vi "S2DS_Scan type change.vi"(10 "All channel parameters":T1 {"Scan parameters"."Y data taking" items=["in both direction", "in up direction only", "in down direction only"]; "Scan parameters"."X data taking" items=["in both direction", "in up direction only", "in down direction only"]}) -> (2 "All channel parameters (out)":T1 {"Scan parameters"."Y data taking" items=["in both direction", "in up direction only", "in down direction only"]; "Scan parameters"."X data taking" items=["in both direction", "in up direction only", "in down direction only"]})   [LabVIEW 2025]
uses:
  TYPE DEFS/S2DS_All Channel Parameters.ctl
  TYPE DEFS/S2DS_WC info.ctl
  TYPE DEFS/S2DS_Single WC info.ctl
  TYPE DEFS/S2DS_RC info.ctl
  TYPE DEFS/S2DS_Single RC info.ctl
  TYPE DEFS/S2DS_DAC info new.ctl
  TYPE DEFS/S2DS_Single DC info.ctl
  TYPE DEFS/S2DS_Array Inst Info.ctl
  TYPE DEFS/S2DS_Sweep Info.ctl
panel:
  out "String":string
  in  "Select Y channel":u16(ring) items=["A", "B"]
  in  "Select X channel":u16(ring) items=["A", "B"]
  in  "stop":bool
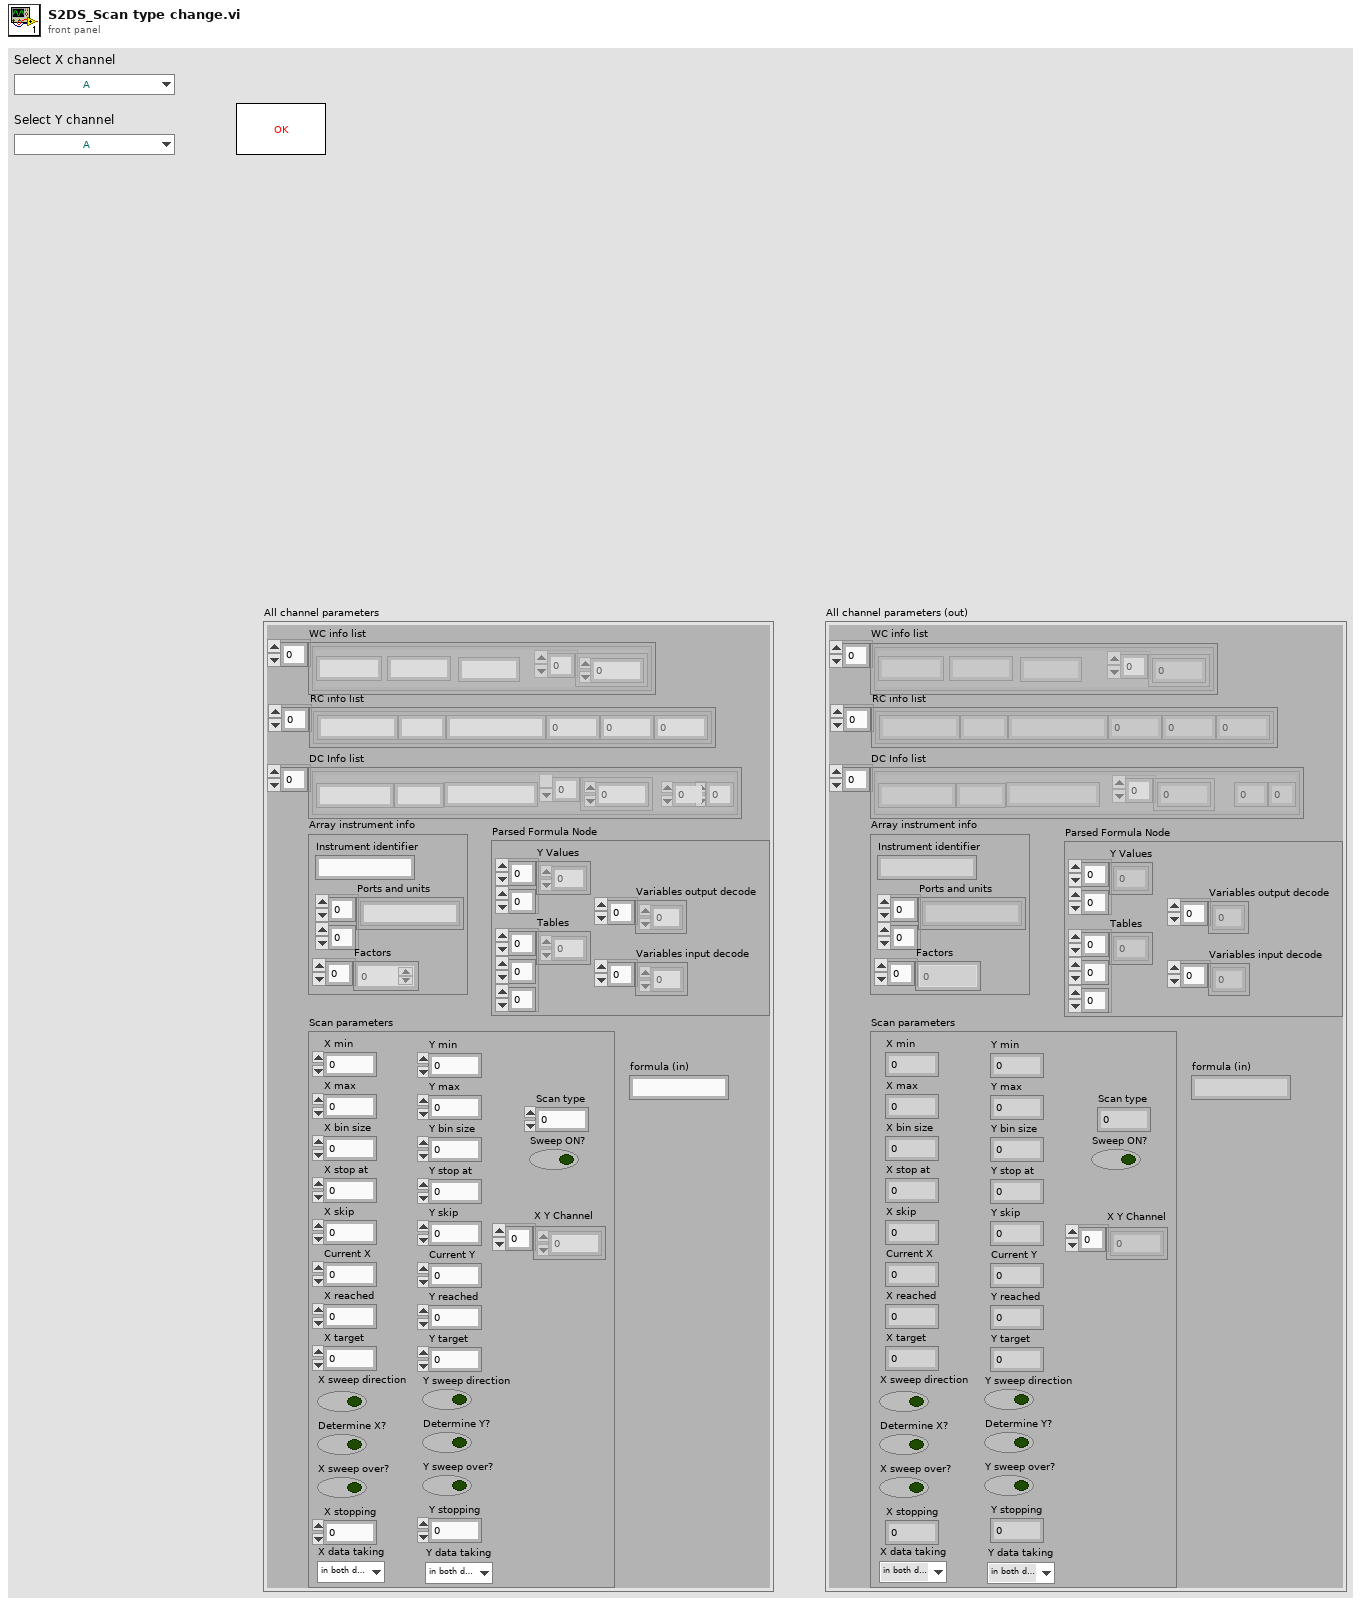
[diagram p1: front panel]
types:
  T1 = typedef "S2DS_All Channel Parameters.ctl" = cluster{"WC info list":T2, "RC info list":T4, "DC Info list":T6, "Array instrument info":T8, "Scan parameters":T9, "Parsed Formula Node":cluster{"Y Values":dbl[][], "Tables":i32[][][], "Variables input decode":i32[], "Variables output decode":i32[]}, "formula (in)":string}
  T2 = typedef "S2DS_WC info.ctl" = T3[]
  T3 = typedef "S2DS_Single WC info.ctl" = cluster{"Instrument identifier":string, "Write channel parameters":dbl[], "Name":string, "Unit":string}
  T4 = typedef "S2DS_RC info.ctl" = T5[]
  T5 = typedef "S2DS_Single RC info.ctl" = cluster{"Instrument identifier":string, "Factor":dbl, "Averaging":i32, "Wait (ms)":i32, "Unit":string, "Name":string}
  T6 = typedef "S2DS_DAC info new.ctl" = T7[]
  T7 = typedef "S2DS_Single DC info.ctl" = cluster{"Operation identifier":string, "DC parameters":dbl[], "U":i32, "V":i32, "Name":string, "Unit":string}
  T8 = typedef "S2DS_Array Inst Info.ctl" = cluster{"Instrument identifier":string, "Ports and units":string[][], "Factors":dbl[]}
  T9 = typedef "S2DS_Sweep Info.ctl" = cluster{"X min":ext, "X max":dbl, "Y min":dbl, "Y max":dbl, "X bin size":dbl, "Y bin size":dbl, "X stop at":dbl, "Y stop at":dbl, "X skip":u64, "Y skip":u64, "Current X":dbl, "Current Y":dbl, "X reached":i32, "Y reached":i32, "X target":dbl, "Y target":dbl, "Sweep ON?":bool, "X sweep direction":bool, "Y sweep direction":bool, "Determine X?":bool, "Determine Y?":bool, "X sweep over?":bool, "Y sweep over?":bool, "Scan type":i32, "X stopping":i32, "Y stopping":i32, "X Y Channel":u16[], "X data taking":u16, "Y data taking":u16}
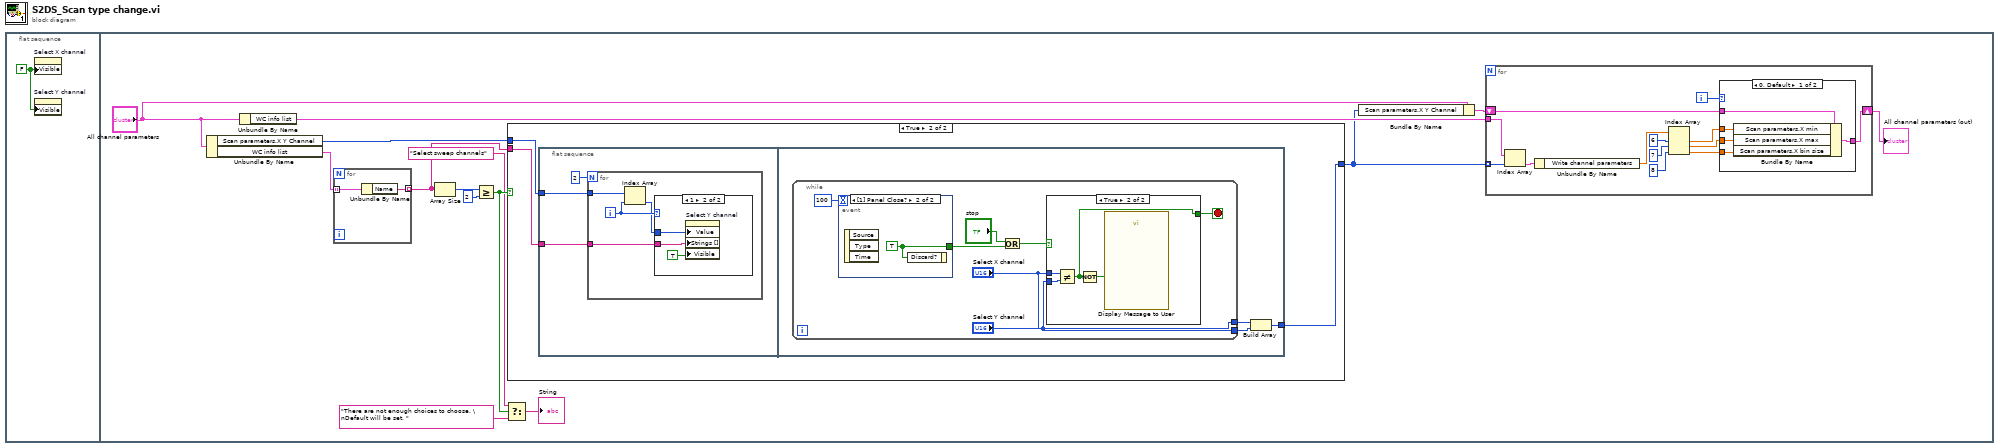
[diagram p0: block diagram]
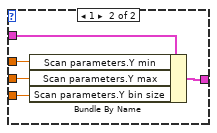
[diagram p2: hidden frame]
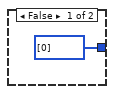
[diagram p3: hidden frame]
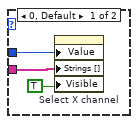
[diagram p4: hidden frame]
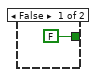
[diagram p5: hidden frame]
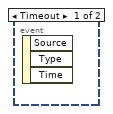
[diagram p6: hidden frame]
diagram:
  n1 = flat-sequence {
    frame #0 {
      w1 = FALSE ("Visible")
      n2 = property on="Select X channel" class="Ring (strict)"("Visible"=w1) -> ()  [unwired: 2 in, 2 out]
      n3 = property on="Select Y channel" class="Ring (strict)"("Visible"=w1) -> ()  [unwired: 2 in, 2 out]
    }
    frame #1 {
      n4 = Unbundle By Name("All channel parameters") -> ("Scan parameters.X Y Channel"=w15:u16[], "WC info list"=w14:T2)
      n5 = Unbundle By Name("All channel parameters") -> ("WC info list"=w5:T2)
      n6 = for {
        tunnel: w14 -> [w73] mode=indexing
        tunnel: [w72] -> w13 mode=indexing
        n7 = Unbundle By Name(w73) -> ("Name"=w72:string)
      }
      n8 = Array Size(array=w13) -> (size(s)=w12:i32)
      n9 = Greater Or Equal?(x=w12, y=2) -> (x >= y?=w10:bool)
      n10 = Select(t="Select sweep channels" ("String"), s=w10, f="There are not enough choices to choose. \nDefault will be set. ") -> (s? t:f=→"String":string)
      n11 = case shown="True" w10 {
        tunnel: w15 -> [_ w42]
        tunnel: w13 -> [_ w41]
        tunnel: [u16[] [0] w40] -> w4
        frame False {
        }
        frame True {
          n12 = flat-sequence {
            tunnel: w42 -> [w45]
            tunnel: w41 -> [w44]
            tunnel: [w56] -> w40
            frame #0 {
              n13 = for {
                N: 2 -> [_]
                tunnel: w45 -> [w48]
                tunnel: w44 -> [w49]
                i -> [w47]
                n14 = Index Array(array=w48, index=w47) -> (element=w46:u16)
                n15 = case shown="1" w47 {
                  tunnel: w46 -> [w52 w55]
                  tunnel: w49 -> [w51 w54]
                  frame 0, Default {
                    n16 = property on="Select X channel" class="Ring (strict)"("Value"=w52, "Strings []"=w51, "Visible"=TRUE) -> ()  [unwired: 2 in, 2 out]
                  }
                  frame 1 {
                    n17 = property on="Select Y channel" class="Ring (strict)"("Value"=w55, "Strings []"=w54, "Visible"=TRUE) -> ()  [unwired: 2 in, 2 out]
                  }
                }
              }
            }
            frame #1 {
              n18 = while {
                tunnel: ["Select Y channel"] -> w57
                tunnel: ["Select X channel"] -> w58
                stop <- w62 stop-if-true
                n19 = event shown="[1] Panel Close?" {
                  selector: _ -> [_ _]
                  dyn-events: _ -> [_ _]
                  timeout: 100 -> [_ _]
                  tunnel: [_ w71] -> w60
                  event Timeout {
                    n20 = event-data() -> ()  [unwired: 1 in, 3 out]
                  }
                  event Panel Close? {
                    w71 = TRUE ("Discard?")
                    n21 = event-data() -> ()  [unwired: 1 in, 3 out]
                    n22 = event-data("Discard?"=w71) -> ()  [unwired: 1 in, 1 out]
                  }
                }
                n23 = Or(x="stop", y=w60) -> (x .or. y?=w59:bool)
                n24 = case shown="True" w59 {
                  tunnel: "Select X channel" -> [_ w70]
                  tunnel: "Select Y channel" -> [_ w69]
                  tunnel: [FALSE w67] -> w62
                  frame False {
                  }
                  frame True {
                    n25 = Not Equal?(x=w70, y=w69) -> (x != y?=w67:bool)
                    n26 = Not(x=w67) -> (.not. x?=w68:bool)
                    n27 = call "Display Message to User"("Enable"=w68) -> ()  [unwired: 9 in, 2 out]
                  }
                }
              }
              n28 = Build Array(w58, w57) -> (w56:u16[])
            }
          }
        }
      }
      n29 = Bundle By Name(cluster="All channel parameters", "Scan parameters.X Y Channel"=w4) -> (w3:T1)
      n30 = for {
        tunnel: w5 -> [w28]
        tunnel: w4 -> [w27] mode=indexing
        shift-right: [w25] -> w2
        shift-left: w3 -> [w26]
        i -> [w24]
        n31 = Index Array(array=w28, index=w27) -> (element=w23:T3)
        n32 = Unbundle By Name(w23) -> ("Write channel parameters"=w22:dbl[])
        n33 = Index Array(array=w22, index #1=6 ("index"), index #2=7 ("index"), index #3=8 ("index")) -> (element #1=w18:dbl, element #2=w17:dbl, element #3=w16:dbl)
        n34 = case shown="0, Default" w24 {
          tunnel: [w32 w37] -> w25
          tunnel: w26 -> [w33 w38]
          tunnel: w18 -> [w31 w36]
          tunnel: w17 -> [w30 w35]
          tunnel: w16 -> [w29 w34]
          frame 0, Default {
            n35 = Bundle By Name(cluster=w33, "Scan parameters.X min"=w31, "Scan parameters.X max"=w30, "Scan parameters.X bin size"=w29) -> (w32:T1)
          }
          frame 1 {
            n36 = Bundle By Name(cluster=w38, "Scan parameters.Y min"=w36, "Scan parameters.Y max"=w35, "Scan parameters.Y bin size"=w34) -> (w37:T1)
          }
        }
      }
      "All channel parameters (out)" <- w2
    }
  }
